vi "Test WS Local Echo Server.vi"(8 "error in (no error)":errorcluster, 11 "TestCase in":refnum<class "Test WebSocket Server.lvclass">) -> (0 "error out":errorcluster, 3 "TestCase out":refnum<class "Test WebSocket Server.lvclass">)   [LabVIEW 2013, in "Test WebSocket Server.lvclass"]
uses:
  Test WebSocket Server.lvclass
  WebSockets/WebSocket Server/WebSocket Server.lvclass
  WebSockets/WebSocket Client/WebSocket Client.lvclass
  <vilib>/addons/_JKI Toolkits/VI Tester/TestCase.llb/TestCase.lvclass
  Sockets/VISA TCP Socket/VISA TCP.lvclass
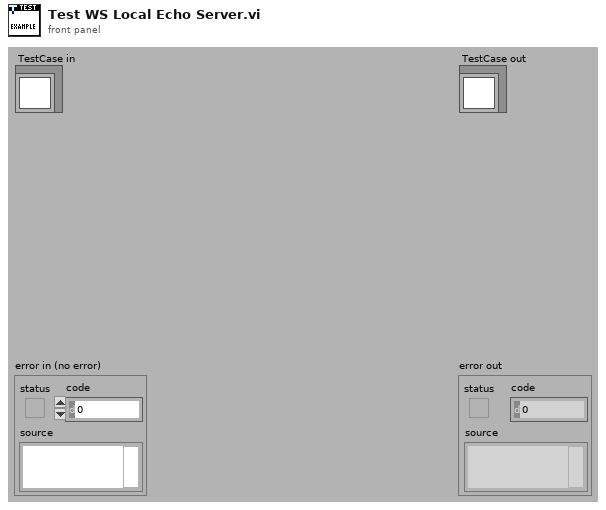
[diagram p1: front panel]
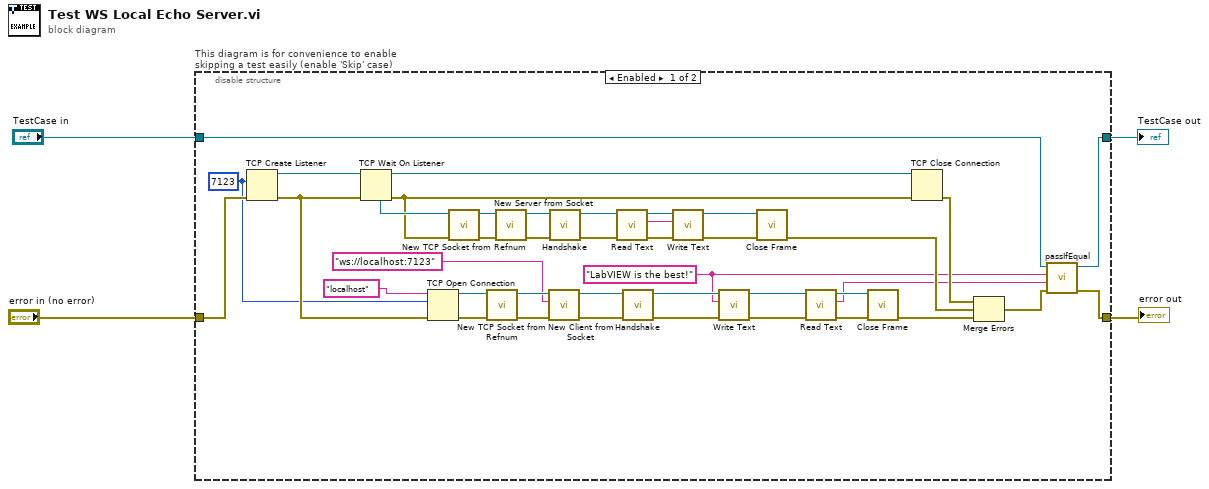
[diagram p0: block diagram]
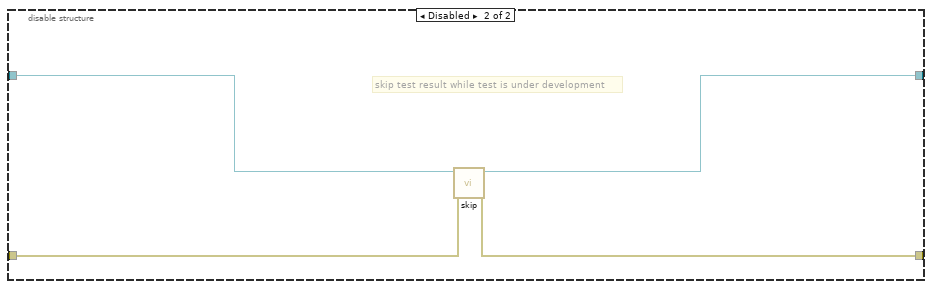
[diagram p2: hidden frame]
diagram:
  n1 = disable-structure "This diagram is for convenience to enable skipping a test easily (enable 'Skip' case)" shown="Enabled" {
    disable-tunnel: "TestCase in" -> [w43 w49]
    disable-tunnel: [w45 w47] -> w1
    disable-tunnel: [w44 w48] -> w3
    disable-tunnel: "error in (no error)" -> [w29 w46]
    frame Enabled {
      w7 = u16 7123 ("port")
      w9 = "LabVIEW is the best!" ("String")
      n2 = TCP Create Listener(8:w29, 10:w7) -> (0:w28:errorcluster, 3:w30:refnum<k5>)  [unwired: 3 in, 1 out]
      n3 = TCP Wait On Listener(8:w28, 11:w30) -> (0:w12:errorcluster, 3:w11:refnum<k5>, 4:w14:refnum<k5>)  [unwired: 2 in, 2 out]
      n4 = TCP Open Connection(address="localhost", remote port or service name=w7, error in (no error)=w28) -> (connection ID=w42:refnum<k5>, error out=w41:errorcluster)  [unwired: 2 in]
      n5 = call "New TCP Socket from Refnum.vi"("error in (no error)"=w12, "TCP Network Connection Refnum"=w14) -> ("error out"=w26:errorcluster, "VISA TCP out"=w27:refnum<class "VISA TCP.lvclass">)  [unwired: 8 in]
      n6 = call "New TCP Socket from Refnum.vi"("error in (no error)"=w41, "TCP Network Connection Refnum"=w42) -> ("error out"=w40:errorcluster, "VISA TCP out"=w39:refnum<class "VISA TCP.lvclass">)  [unwired: 8 in]
      n7 = call "New Server from Socket.vi"("error in (no error)"=w26, "Socket"=w27) -> ("error out"=w25:errorcluster, "WebSocket Server out"=w24:refnum<class "WebSocket Server.lvclass">)  [unwired: 8 in]
      n8 = call "New Client from Socket.vi"("error in (no error)"=w40, "WebSocket URL"="ws://localhost:7123" ("address"), "Socket in"=w39) -> ("error out"=w38:errorcluster, "WebSocket Client out"=w37:refnum<class "WebSocket Client.lvclass">)  [unwired: 7 in]
      n9 = call-dynamic "Handshake.vi"("error in (no error)"=w25, "WebSocket Connection in"=w24) -> ("error out"=w23:errorcluster, "WebSocket Connection out"=w22:refnum<class "WebSocket Server.lvclass">)  [unwired: 8 in]
      n10 = call-dynamic "Read Text.vi"("error in (no error)"=w23, "WebSocket in"=w22) -> ("error out"=w21:errorcluster, "Data"=w19:string, "WebSocket out"=w20:refnum<class "WebSocket Server.lvclass">)  [unwired: 7 in]
      n11 = call-dynamic "Handshake.vi"("error in (no error)"=w38, "WebSocket Client in"=w37) -> ("error out"=w36:errorcluster, "WebSocket Client out"=w35:refnum<class "WebSocket Client.lvclass">)  [unwired: 8 in]
      n12 = call-dynamic "Write Text.vi"("error in (no error)"=w21, "String Data"=w19, "WebSocket in"=w20) -> ("error out"=w18:errorcluster, "WebSocket out"=w17:refnum<class "WebSocket Server.lvclass">)  [unwired: 7 in]
      n13 = call-dynamic "Write Text.vi"("error in (no error)"=w36, "String Data"=w9, "WebSocket in"=w35) -> ("error out"=w31:errorcluster, "WebSocket out"=w32:refnum<class "WebSocket Client.lvclass">)  [unwired: 7 in]
      n14 = call-dynamic "Close Frame.vi"("error in (no error)"=w18, "WebSockets in"=w17) -> ("error out"=w15:errorcluster)  [unwired: 8 in, 1 out]
      n15 = call-dynamic "Read Text.vi"("error in (no error)"=w31, "WebSocket in"=w32) -> ("error out"=w34:errorcluster, "Data"=w8:string, "WebSocket out"=w33:refnum<class "WebSocket Client.lvclass">)  [unwired: 7 in]
      n16 = call-dynamic "Close Frame.vi"("error in (no error)"=w34, "WebSockets in"=w33) -> ("error out"=w16:errorcluster)  [unwired: 8 in, 1 out]
      n17 = TCP Close Connection(connection ID=w11, error in (no error)=w12) -> (error out=w13:errorcluster)  [unwired: 1 in, 1 out]
      n18 = Merge Errors(w13, w15, w16) -> (w10:errorcluster)
      n19 = call-dynamic "passIfEqual.vi"("error in (no error)"=w10, "y"=w8, "x"=w9, "TestCase in"=w43) -> ("error out"=w44:errorcluster, "TestCase out"=w45:refnum<class "Test WebSocket Server.lvclass">)  [unwired: 6 in]
    }
    frame Disabled {
      # "skip test result while test is under development"
      n20 = call <vilib>:"skip.vi"("error in (no error)"=w46, "TestCase in"=w49) -> ("error out"=w48:errorcluster, "TestCase out"=w47:refnum<class "Test WebSocket Server.lvclass">)  [unwired: 8 in]
    }
  }
  "error out" <- w3
  "TestCase out" <- w1
